vi "EnumAnyBuilderFromMetadata.vi"() -> ()   [LabVIEW 2019]
uses:
  labview source/gRPC lv Support/Shared/Any.ctl
  labview source/gRPC lv Support/Server API/typeDefs/Message Metadata.ctl
  labview source/gRPC lv Support/Server API/typeDefs/Message Element Metadata.ctl
  labview source/gRPC lv Support/Server API/typeDefs/Message Element Type.ctl
  50cd6ca9-b915-40c5-a5da-5a0bdd109e0e.vi
  b9ed661b-4002-4d98-860f-0e3cbd5bf3a1.vi
  8f5c9cc0-1363-4dd4-ad5e-2067650e9c9f.vi
  1a12c270-2529-48ab-8650-0ad34f8ed4bc.vi
  79bcfed6-c06a-4154-86a9-8554a85b91ac.vi
  65d46b58-227a-49f8-b739-8ba8c807fa65.vi
  labview source/gRPC lv Support/Server API/Translate Protobuf Error.vi
  <vilib>/AdvancedString/1D String Array to Delimited String.vi
  labview source/gRPC lv Support/Server API/Server/Get Server DLL Path.vi
  labview source/gRPC lv Support/grpc-lvsupport.lvlib
panel:
  out "Got Expected InvalidEnum Error?":bool
  out "Array":enum32{"a", "b", "c"}[](array[ring])
  out "Enum":enum32{"a", "b", "c"}(ring)
  out "error out":errorcluster
  out "Numeric 2":i32
  out "Any":T1
  out "Numeric":i32
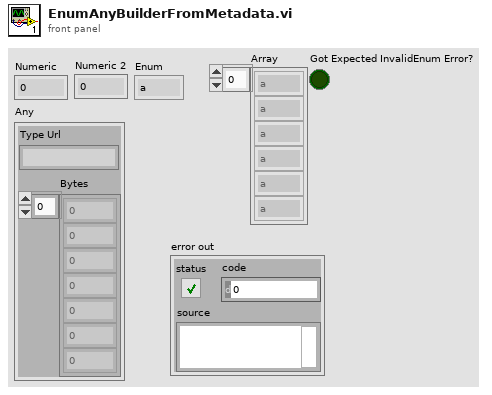
[diagram p1: front panel]
types:
  T1 = typedef "grpc-lvsupport.lvlib/Any.ctl" = cluster{"Type Url":string, "Bytes":u8[]}
  T2 = typedef "grpc-lvsupport.lvlib/Message Element Type.ctl" = enum32{"Int32Value", "FloatValue", "DoubleValue", "BoolValue", "StringValue", "MessageValue", "Int64Value", "UInt32Value", "UInt64Value", "EnumValue", "Bytes", "Fixed64", "Fixed32", "SFixed64", "SFixed32", "SInt64", "SInt32"}
  T3 = typedef "grpc-lvsupport.lvlib/Message Element Metadata.ctl" = cluster{"Field Name":string, "Embedded Message Name":string, "Protobuf Index":i32, "MessageElementType":T2, "Repeated":bool, "Is in Oneof":bool, "Oneof Container Name":string}
  T4 = typedef "grpc-lvsupport.lvlib/Message Metadata.ctl" = cluster{"Version":i32, "Name":string, "Type Url":string, "Elements":T3[], "Has Oneof":bool}
  T5 = typedef "grpc-lvsupport.lvlib/Enum Metadata.ctl" = cluster{"Version":i32, "Name":string, "Type Url":string, "Enum Values":string, "Allow Alias":bool}
  T6 = typedef "grpc-lvsupport.lvlib/grpcId.ctl" = u64
  T7 = cluster{i32, i32, enum32{"a", "b", "c"}, enum32{"a", "b", "c"}[]}
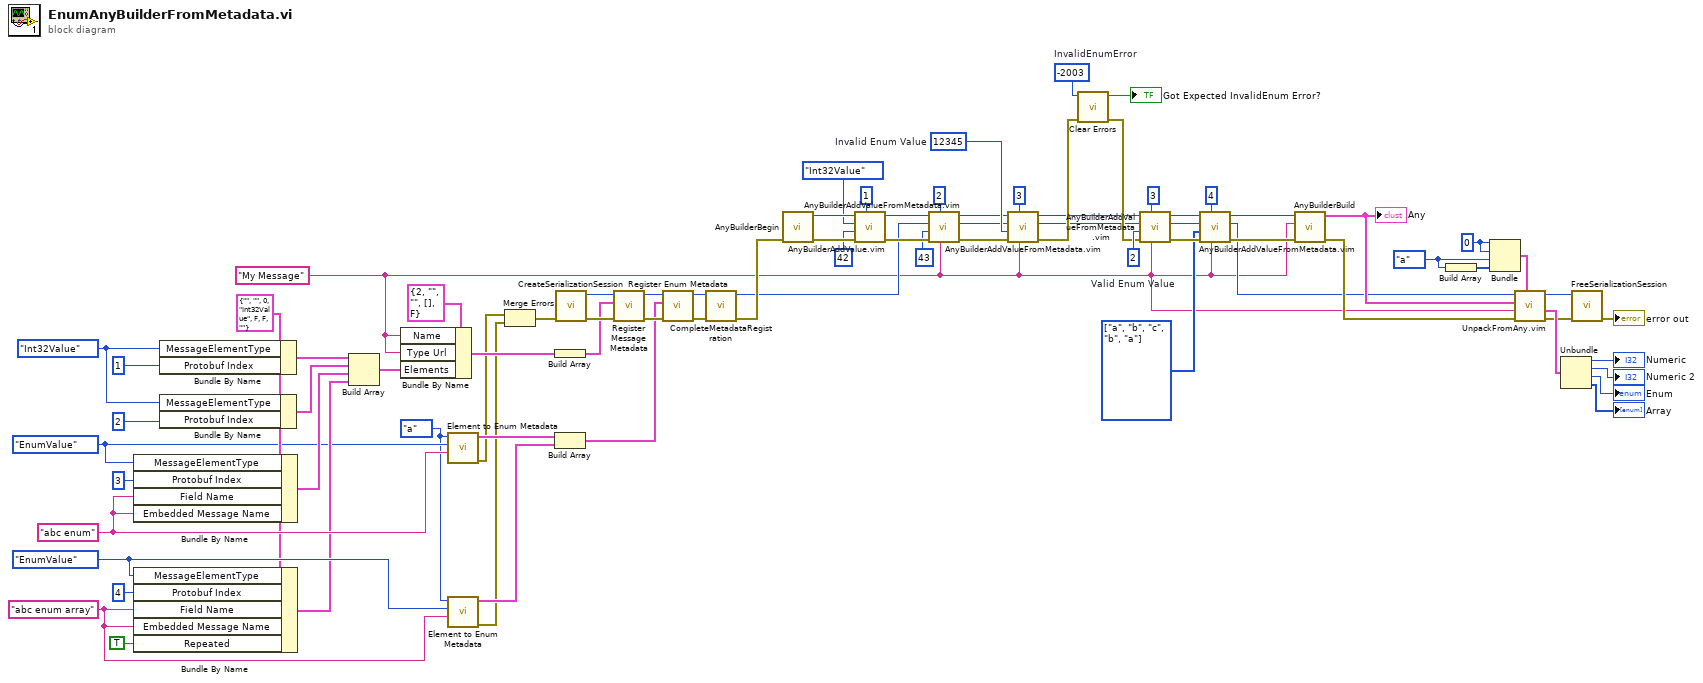
[diagram p0: block diagram]
diagram:
  w11 = -2003  # InvalidEnumError
  w14 = 12345  # Invalid Enum Value
  w23 = enum32{"a", "b", "c"}[] [enum."a", enum."b", enum."c", enum."b", enum."a"] items=["a", "b", "c"]
  w36 = Message_Element_Type."EnumValue" ("MessageElementType")
  w35 = "abc enum array" ("Embedded Message Name")
  w21 = enum32{"a", "b", "c"}."a"
  w18 = 2  # Valid Enum Value
  w42 = 0
  w50 = Message_Element_Type."Int32Value" ("MessageElementType")
  w29 = Message_Element_Type."EnumValue" ("MessageElementType")
  w46 = "abc enum" ("Embedded Message Name")
  w31 = T3 {"Field Name"="", "Embedded Message Name"="", "Protobuf Index"=0, "MessageElementType"=enum."Int32Value", "Repeated"=FALSE, "Is in Oneof"=FALSE, "Oneof Container Name"=""} ("MessageElementMetadata")
  w19 = enum32{"a", "b", "c"}."a"
  w7 = "My Message" ("Message Type")
  n1 = Bundle By Name(cluster=w31, "MessageElementType"=w29, "Protobuf Index"=3, "Field Name"=w46, "Embedded Message Name"=w46) -> (w52:T3)
  n2 = Bundle By Name(cluster=w31, "MessageElementType"=w36, "Protobuf Index"=4, "Field Name"=w35, "Embedded Message Name"=w35, "Repeated"=TRUE) -> (w30:T3)
  n3 = Bundle By Name(cluster=w31, "MessageElementType"=w50, "Protobuf Index"=1) -> (w39:T3)
  n4 = Bundle By Name(cluster=w31, "MessageElementType"=w50, "Protobuf Index"=2) -> (w44:T3)
  n5 = Build Array(w39, w44, w52, w30) -> (w55:T3[])
  n6 = Bundle By Name(cluster=T4 {"Version"=2, "Name"="", "Type Url"="", "Elements"=[], "Has Oneof"=FALSE} ("Message Metadata"), "Name"=w7, "Type Url"=w7, "Elements"=w55) -> (w54:T4)
  n7 = call "Element to Enum Metadata.vi"("Name"=w46, "MessageElementType"=w29, "Element"=w19) -> ("error out"=w34:errorcluster, "Enum Metadata"=w45:T5)  [unwired: 6 in, 1 out]
  n8 = call "Element to Enum Metadata.vi"("Name"=w35, "MessageElementType"=w36, "Element"=w19) -> ("error out"=w33:errorcluster, "Enum Metadata"=w37:T5)  [unwired: 6 in, 1 out]
  n9 = Merge Errors(w34, w33) -> (w32:errorcluster)
  n10 = Build Array(w54) -> (w53:T4[])
  n11 = Build Array(w45, w37) -> (w47:T5[])
  n12 = call "CreateSerializationSession.vi"("error in"=w32) -> ("error out"=w66:errorcluster, "Serialization Session ID"=w76:T6)  [unwired: 9 in]
  n13 = call "Register Message Metadata.vi"("error in"=w66, "Messages"=w53, "gRPCid in"=w76) -> ("error out"=w62:errorcluster, "gRPCid out"=w61:T6)  [unwired: 7 in]
  n14 = call "Register Enum Metadata.vi"("error in"=w62, "Enum Metadata"=w47, "gRPCid in"=w61) -> ("error out"=w59:errorcluster, "gRPCid out"=w60:T6)  [unwired: 7 in]
  n15 = call "CompleteMetadataRegistration.vi"("error in"=w59, "gRPC ID in"=w60) -> ("error out"=w58:errorcluster, "gRPC ID Out"=w40:T6)  [unwired: 8 in]
  n16 = call "AnyBuilderBegin.vi"("error in"=w58) -> ("error out"=w68:errorcluster, "Builder Ref Out"=w79:T6)  [unwired: 8 in]
  n17 = call "AnyBuilderAddValue.vim"("protobufId"=1, "error in"=w68, "Value"=42, "MessageElementType"=Message_Element_Type."Int32Value", "gRPCid in"=w79) -> ("error out"=w67:errorcluster, "gRPCid out"=w71:u64)  [unwired: 5 in]
  n18 = call "AnyBuilderAddValueFromMetadata.vim"("message type"=w7, "protobufId"=2, "error in"=w67, "Value"=43, "metadata owner id"=w40, "builderId in"=w71) -> ("error out"=w6:errorcluster, "metadata owner id out"=w5:u64, "builderId out"=w4:u64)  [unwired: 3 in]
  n19 = call "AnyBuilderAddValueFromMetadata.vim"("message type"=w7, "protobufId"=3, "error in"=w6, "Value"=w14, "metadata owner id"=w5, "builderId in"=w4) -> ("error out"=w13:errorcluster, "metadata owner id out"=w1:u64, "builderId out"=w2:u64)  [unwired: 3 in]
  n20 = call <vilib>:"Clear Errors.vi"("error in (no error)"=w13, "specific error code to clear (0: all)"=w11) -> ("error out"=w3:errorcluster, "specific error cleared?"=→"Got Expected InvalidEnum Error?":bool)  [unwired: 4 in]
  n21 = call "AnyBuilderAddValueFromMetadata.vim"("message type"=w7, "protobufId"=3, "error in"=w3, "Value"=w18, "metadata owner id"=w1, "builderId in"=w2) -> ("error out"=w27:errorcluster, "metadata owner id out"=w25:u64, "builderId out"=w28:u64)  [unwired: 3 in]
  n22 = call "AnyBuilderAddValueFromMetadata.vim"("message type"=w7, "protobufId"=4, "error in"=w27, "Value"=w23, "metadata owner id"=w25, "builderId in"=w28) -> ("error out"=w10:errorcluster, "metadata owner id out"=w8:u64, "builderId out"=w9:u64)  [unwired: 3 in]
  n23 = call "AnyBuilderBuild.vi"("error in"=w10, "Message Type"=w7, "Builder Ref"=w9) -> ("error out"=w57:errorcluster, "Any"=w75:T1)  [unwired: 7 in]
  "Any" <- w75
  n24 = Build Array(w21) -> (w22:enum32{"a", "b", "c"}[])
  n25 = Bundle(w42, w42, w21, w22) -> (w41:T7)  [unwired: 1 in]
  n26 = call "UnpackFromAny.vim"("Data Type"=w41, "error in"=w57, "Message Type"=w7, "Any"=w75, "gRPCid in"=w8) -> ("error out"=w65:errorcluster, "Unpacked Value"=w74:T7, "gRPCid out"=w72:u64)  [unwired: 4 in]
  n27 = Unbundle(w74) -> (→"Numeric":i32, →"Numeric 2":i32, →"Enum":enum32{"a", "b", "c"}, →"Array":enum32{"a", "b", "c"}[])
  n28 = call "FreeSerializationSession.vi"("error in"=w65, "Serialization Session ID"=w72) -> ("error out"=→"error out":errorcluster)  [unwired: 9 in]
